vi "FTW-CodeGen-DisplayName.vi"(0 "State In":T1) -> (4 "Name":string)   [LabVIEW 2014, in "FTW-Sync-Synchronizer.xnode"]
uses:
  FTW-Sync-Synchronizer.xnode
  FTW-CodeGen-State.ctl
panel:
  # "Inputs"
  # "Outputs"
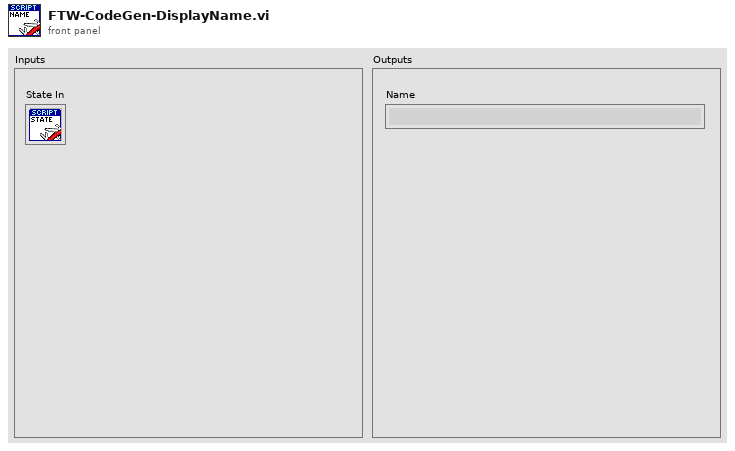
[diagram p1: front panel]
types:
  T1 = typedef "FTW-Sync-Synchronizer.xnode/FTW-CodeGen-State.ctl" = cluster{"InputTerminals":cluster{"Wired?":bool, "ID":string, "DataName":string, "DataColor":u32, "Type":variant}[], "EnableTiming?":bool}
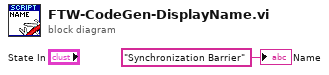
[diagram p0: block diagram]
diagram:
  "Name" <- "Synchronization Barrier" ("Name")
